vi "Unpack AI Values.vi"(9 "Resolution":u8, 10 "Values":u8[](array[numeric])) -> (2 "ADC Ticks":u32[](array[numeric]))   [LabVIEW 2020, in "Device.lvlib"]
uses:
  Device.lvlib
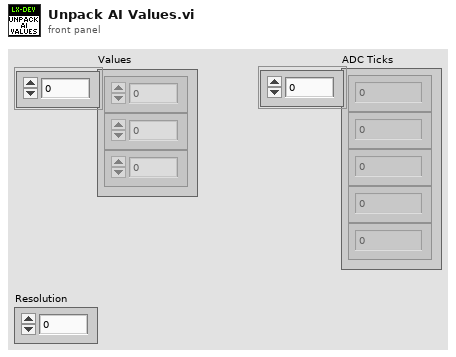
[diagram p1: front panel]
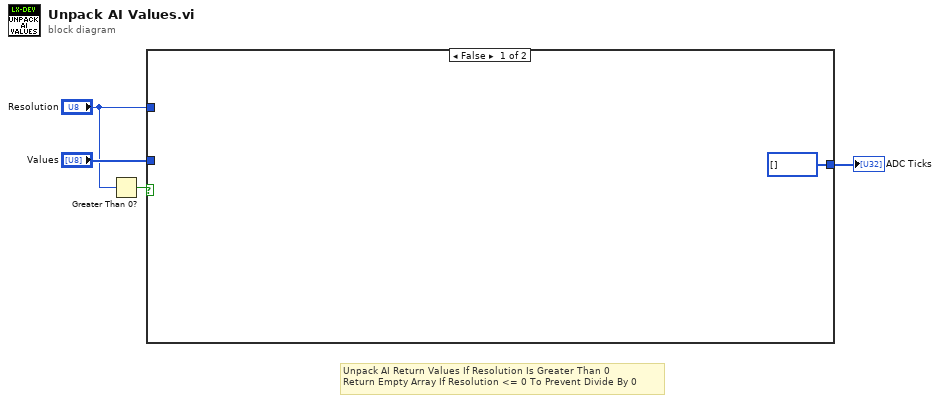
[diagram p0: block diagram]
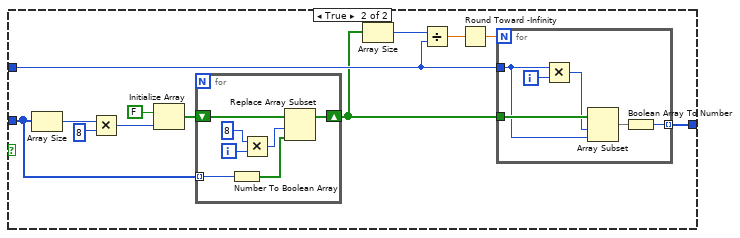
[diagram p2: hidden frame]
diagram:
  # "Unpack AI Return Values If Resolution Is Greater Than 0\nReturn Empty Array If Resolution <= 0 To Prevent Divide By 0"
  n1 = Greater Than 0?(x="Resolution") -> (x > 0?=w2:bool)
  n2 = case shown="False" w2 {
    tunnel: "Values" -> [_ w17]
    tunnel: "Resolution" -> [_ w10]
    tunnel: [u32[] [] w9] -> w4
    frame False {
    }
    frame True {
      n3 = Array Size(array=w17) -> (size(s)=w15:i32)
      n4 = Multiply(x=w15, y=8) -> (x*y=w14:i32)
      n5 = Initialize Array(FALSE, w14) -> (w12:bool[])
      n6 = for {
        tunnel: w17 -> [w30] mode=indexing
        shift-right: [w29] -> w6
        shift-left: w12 -> [w25]
        i -> [w28]
        n7 = Number To Boolean Array(number=w30) -> (Boolean array=w24:bool[])
        n8 = Multiply(x=8, y=w28) -> (x*y=w26:i32)
        n9 = Replace Array Subset(array=w25, new element=w24, index=w26) -> (w29:bool[])
      }
      n10 = Array Size(array=w6) -> (size(s)=w11:i32)
      n11 = Divide(x=w11, y=w10) -> (x/y=w8:dbl)
      n12 = Round Toward -Infinity(1:w8) -> (0:w7:dbl)
      n13 = for {
        N: w7 -> [_]
        tunnel: w6 -> [w23]
        tunnel: w10 -> [w20]
        tunnel: [w18] -> w9 mode=indexing
        i -> [w22]
        n14 = Multiply(x=w20, y=w22) -> (x*y=w21:i32)
        n15 = Array Subset(array=w23, index=w21, length=w20) -> (w19:bool[])
        n16 = Boolean Array To Number(Boolean array=w19) -> (number=w18:u32)
      }
    }
  }
  "ADC Ticks" <- w4
